vi "GetEvtSignal.vi"(8 "error in (no error)":errorcluster, 11 "C37EventPlugin in":refnum<class "C37Plugin.lvclass">) -> (0 "error out":errorcluster, 3 "C37EventPlugin out":refnum<class "C37Plugin.lvclass">)   [LabVIEW 2014, in "WfrmPlugins.lvlib" / "C37Plugin.lvclass"]
uses:
  C37Plugin.lvclass
  EventPluginBaseClass/BaseWfrmPlugin.lvclass/BaseWfrmPlugin.ctl
  EventPluginBaseClass/Accessors/Read EndTime.vi
  <vilib>/imath/engines/lvmath2/RunTimeEngine/IndexRead/NIMS V(S).vi
  <instcachedir>/0/NIMS V(S)_0488751826AF41519A22953C041130DC.lvgen/NIMS V(S)_0488751826AF41519A22953C041130DC_000.vi
  <vilib>/imathl/engines/lvmath/Functions/Error Handling/Create Error.vi
  <vilib>/imath/engines/lvmath2/RunTimeEngine/RangeToken/NIMS_Range.vi
  <instcachedir>/0/NIMS_Range_9BCE657718DF4976A877346C61F22738.lvgen/NIMS_Range_9BCE657718DF4976A877346C61F22738_000.vi
  C:/Labview Data/MathScriptVIs/MCStatic_33564263232_24a1c065333935aa4738809c0966bb17.vi
  <instcachedir>/0/MCStatic_33564263232_24a1c065333935aa4738809c0966bb17_7201A64FCC71402282BEAA67FEE2504E.lvgen/MCStatic_33564263232_24a1c065333935aa4738809c0966bb17_7201A64FCC71402282BEAA67FEE2504E_000.vi
  <vilib>/imath/engines/lvmath2/RunTimeEngine/NodeEndStatement/NIMS_NodeEndStatement_Output.vi
  <instcachedir>/0/NIMS_NodeEndStatement_Output_53EC0D466D134D7ABD903AC30B43404B.lvgen/NIMS_NodeEndStatement_Output_53EC0D466D134D7ABD903AC30B43404B_002.vi
  <vilib>/imath/engines/lvmath2/RunTimeEngine/ErrorHandling/NIMS_Finalize Error.vi
  Matlab/C37/genC37Signal.m
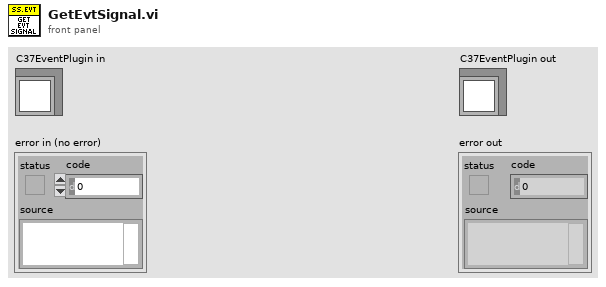
[diagram p1: front panel]
types:
  T1 = typedef "WfrmPlugins.lvlib/BaseWfrmPlugin.lvclass/WfrmConfig.ctl" = cluster{"T0(UTC)":dbl, "F0":dbl, "Fs":i32, "FSamp":u32}
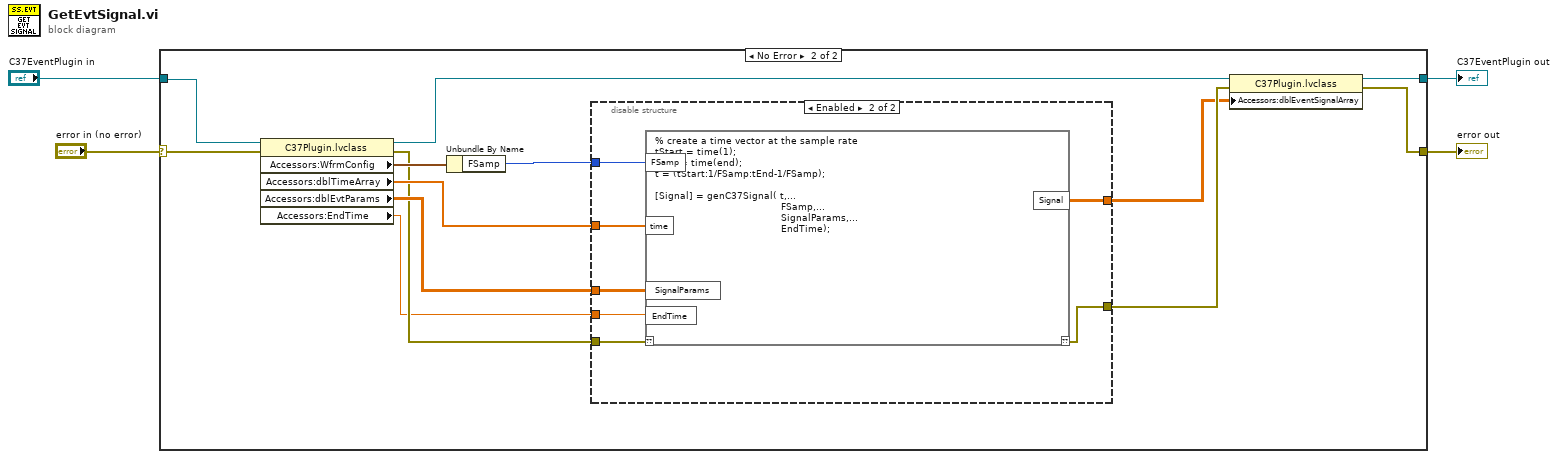
[diagram p0: block diagram]
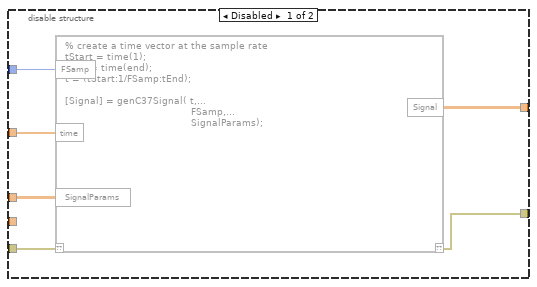
[diagram p3: hidden frame]
diagram:
  n1 = case shown="No Error" "error in (no error)" {
    selector: "error in (no error)" -> [w6 w16]
    tunnel: [w5 w19] -> w4
    tunnel: "C37EventPlugin in" -> [w5 w17]
    tunnel: [w6 w18] -> w3
    frame Error {
    }
    frame No Error {
      n2 = property class="C37Plugin.lvclass"(reference=w17, error in=w16) -> (reference out=w13:refnum<class "C37Plugin.lvclass">, error out=w9:errorcluster, "Accessors:WfrmConfig"=w15:T1, "Accessors:dblTimeArray"=w11:dbl[], "Accessors:dblEvtParams"=w10:dbl[][], "Accessors:EndTime"=w7:dbl)
      n3 = Unbundle By Name(w15) -> ("FSamp"=w14:u32)
      n4 = disable-structure shown="Enabled" {
        disable-tunnel: w14 -> [w25 w32]
        disable-tunnel: [w24 w27] -> w12
        disable-tunnel: w11 -> [w23 w31]
        disable-tunnel: w10 -> [w22 w30]
        disable-tunnel: w9 -> [w21 w29]
        disable-tunnel: [w20 w28] -> w8
        disable-tunnel: w7 -> [_ w26]
        frame Disabled {
          n5 = script code="% create a time vector at the sample rate\ntStart = time(1);\ntEnd = time(end);\nt = (tStart:1/FSamp:tEnd);\n\n[Signal] = genC37Signal( t,...\n                                          FSamp,...\n                                          SignalParams);"("??"=w21, "FSamp"=w25, "time"=w23, "SignalParams"=w22) -> ("??"=w24:errorcluster, "Signal"=w20:dbl[][])
        }
        frame Enabled {
          n6 = mathscript code="% create a time vector at the sample rate\ntStart = time(1);\ntEnd = time(end);\nt = (tStart:1/FSamp:tEnd-1/FSamp);\n\n[Signal] = genC37Signal( t,...\n                                          FSamp,...\n                                          SignalParams,...\n                                          EndTime);"("??"=w29, "FSamp"=w32, "time"=w31, "SignalParams"=w30, "EndTime"=w26) -> ("??"=w27:errorcluster, "Signal"=w28:dbl[][])
        }
      }
      n7 = property class="C37Plugin.lvclass"(reference=w13, error in=w12, "Accessors:dblEventSignalArray"=w8) -> (reference out=w19:refnum<class "C37Plugin.lvclass">, error out=w18:errorcluster)
    }
  }
  "error out" <- w3
  "C37EventPlugin out" <- w4
